vi "PXI-Init Counter Params.vi"(11 "error in":errorcluster) -> (8 "Counter Parameters":T1={"Counter"="PXI1Slot4/ctr0", "Hi ticks"=5, "Low ticks"=4995, "Idle state"=10214, "Delay ticks"=0} {"Idle state" items=["High"=10192, "Low"=10214]; "Low ticks" max=1}, 15 "error out":errorcluster)   [LabVIEW 2015]
uses:
  PXI Key Wrapper VIs/PXI-Read Key Wrapper (I32).vi
panel:
  in  "Dummy Counter Struct":T1={"Counter"="PXI1Slot4/ctr0", "Hi ticks"=0, "Low ticks"=0, "Idle state"=10214, "Delay ticks"=0} {"Idle state" items=["High"=10192, "Low"=10214]; "Low ticks" max=1}
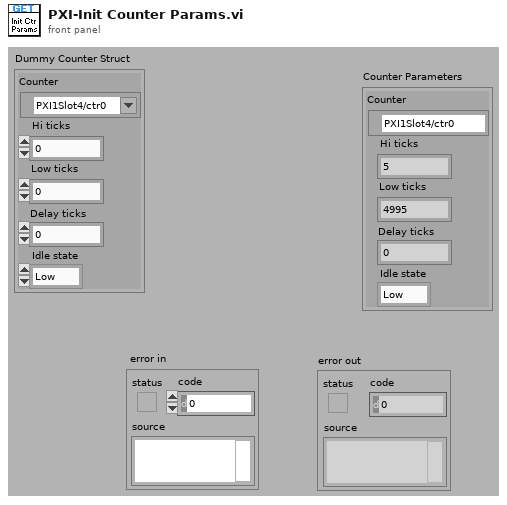
[diagram p1: front panel]
types:
  T1 = cluster{"Counter":tag, "Hi ticks":u32, "Low ticks":u32, "Idle state":i32, "Delay ticks":u32}
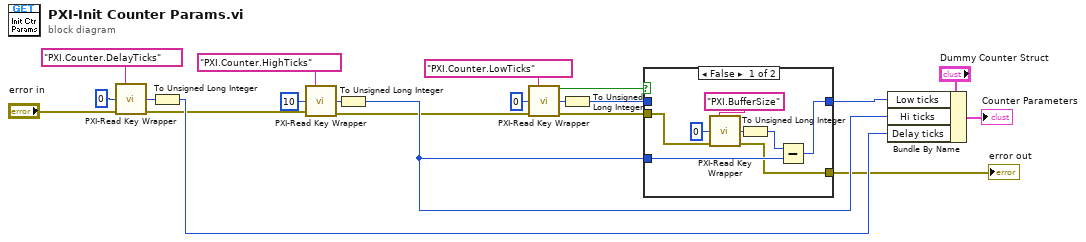
[diagram p0: block diagram]
diagram:
  n1 = call-poly "PXI-Read Key Wrapper.vi"("key"="PXI.Counter.DelayTicks" ("string"), "default value"=0, "error in (no error)"="error in") -> ("value"=w11:i32, "error out"=w3:errorcluster)  [unwired: 10 in, 1 out]
  n2 = To Unsigned Long Integer(number=w11) -> (unsigned 32bit integer=w4:u32)
  n3 = call-poly "PXI-Read Key Wrapper.vi"("key"="PXI.Counter.HighTicks" ("string"), "default value"=10, "error in (no error)"=w3) -> ("value"=w17:i32, "error out"=w5:errorcluster)  [unwired: 10 in, 1 out]
  n4 = To Unsigned Long Integer(number=w17) -> (unsigned 32bit integer=w6:u32)
  n5 = call-poly "PXI-Read Key Wrapper.vi"("key"="PXI.Counter.LowTicks" ("string"), "default value"=0, "error in (no error)"=w5) -> ("found?"=w7:bool, "value"=w14:i32, "error out"=w2:errorcluster)  [unwired: 10 in]
  n6 = To Unsigned Long Integer(number=w14) -> (unsigned 32bit integer=w10:u32)
  n7 = case shown="False" w7 {
    tunnel: w6 -> [w26 _]
    tunnel: w10 -> [_ w31]
    tunnel: [w24 w31] -> w9
    tunnel: w2 -> [w23 w30]
    tunnel: [w22 w30] -> w1
    frame False {
      n8 = call-poly "PXI-Read Key Wrapper.vi"("key"="PXI.BufferSize" ("string"), "default value"=0, "error in (no error)"=w23) -> ("value"=w29:i32, "error out"=w22:errorcluster)  [unwired: 10 in, 1 out]
      n9 = To Unsigned Long Integer(number=w29) -> (unsigned 32bit integer=w25:u32)
      n10 = Subtract(x=w25, y=w26) -> (x-y=w24:u32)
    }
    frame True {
    }
  }
  "error out" <- w1
  n11 = Bundle By Name(cluster="Dummy Counter Struct", "Low ticks"=w9, "Hi ticks"=w6, "Delay ticks"=w4) -> (→"Counter Parameters":T1)
